vi "Read Analogue.vi"(8 "error in (no error)":errorcluster, 11 "NI Thermo in":refnum<class "NI Thermo.lvclass">) -> (0 "error out":errorcluster, 2 "Waveforms":waveform(dbl)[](array[waveform]), 3 "NI Thermo out":refnum<class "NI Thermo.lvclass">)   [LabVIEW 2025, in "Thermo.lvlib" / "NI Thermo.lvclass"]
uses:
  NI Thermo.lvclass
  NI Thermo.lvclass/NI Thermo.ctl
  Thermo Channel/Thermo Channel.lvclass
  Thermo Channel configuration/Thermo Channel configuration.lvclass
  <vilib>/DAQmx/read.llb/DAQmx Read (Analog 1D DBL NChan 1Samp).vi
  Users/Public/Documents/Sandia National Labs/TSS Plugin/Abstract Engine.lvlibp/Abstract Instrument/Channel.ctl
  Users/Public/Documents/Sandia National Labs/TSS Plugin/Abstract Engine.lvlibp/Abstract Instrument/Abstract Instrument.lvclass
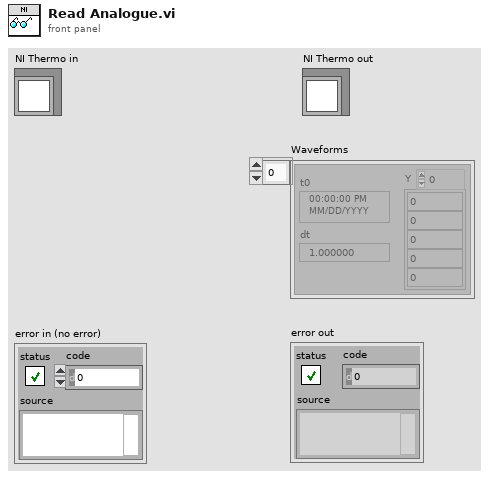
[diagram p1: front panel]
types:
  T1 = typedef "Abstract Engine.lvlibp/Abstract Instrument.lvclass/Channel.ctl" = cluster{"Alias":string, "DataType":enum16{"Anaolg Input", "Waveform"}, "Unit":enum16{"---", "V", "A", "Ohm", "Hz", "uF", "degC", "deg"}, "Upper limit":dbl, "Lower limit":dbl, "Measurement":variant}
  T2 = enum16{"---", "V", "A", "Ohm", "Hz", "uF", "degC", "deg"}
  T3 = typedef "Abstract Engine.lvlibp/Channel configuration.lvclass/Default Channel.ctl" = cluster{"Address":string, "SW Alias":string, "Enabled":bool, "Type":string, "Description":string}
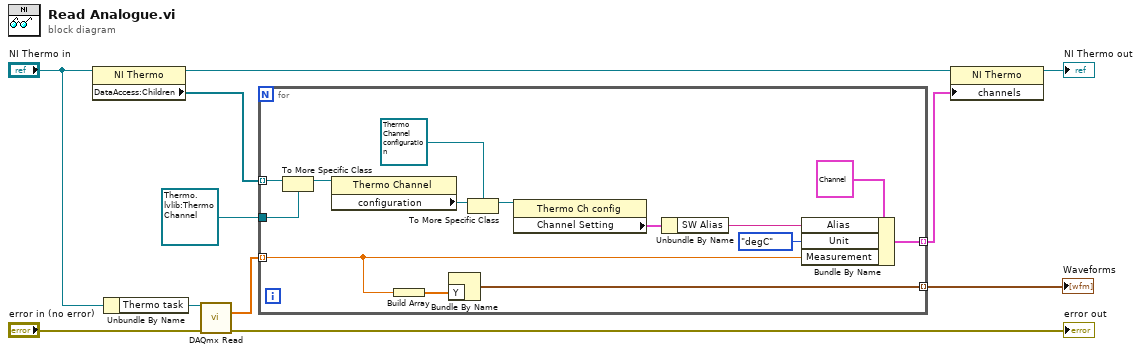
[diagram p0: block diagram]
diagram:
  n1 = property class="NI Thermo"(reference="NI Thermo in") -> (reference out=w7:refnum<class "NI Thermo.lvclass">, "DataAccess:Children"=w6:refnum<data-value>[])  [unwired: 1 in, 1 out]
  n2 = Unbundle By Name("NI Thermo in") -> ("Thermo task"=w8:refnum<k21>)
  n3 = call-poly <vilib>:"DAQmx Read.vi"("task/channels in"=w8, "error in"="error in (no error)") -> ("data"=w4:dbl[], "error out"=→"error out":errorcluster)  [unwired: 11 in, 1 out]
  n4 = for {
    tunnel: w4 -> [w14] mode=indexing
    tunnel: w6 -> [w25] mode=indexing
    tunnel: [w19] -> w2 mode=indexing
    tunnel: refnum<data-value> refnum ("data value reference") -> [w18]
    tunnel: [w12] -> w1 mode=indexing
    n5 = To More Specific Class(target class=w18, reference=w25) -> (specific class reference=w24:refnum<data-value>)  [unwired: 1 in, 1 out]
    n6 = property class="Thermo Channel"(reference=w24) -> ("configuration"=w23:refnum<class "CEF_serializable configuration.lvclass">)  [unwired: 1 in, 2 out]
    n7 = Build Array(w14) -> (w13:dbl[])
    n8 = Bundle By Name("Y"=w13) -> (w12:waveform(dbl))  [unwired: 1 in]
    n9 = To More Specific Class(target class=refnum<class "Thermo Channel configuration.lvclass"> refnum ("Thermo.lvlib:Thermo Ch config"), reference=w23) -> (specific class reference=w22:refnum<class "Thermo Channel configuration.lvclass">)  [unwired: 1 in, 1 out]
    n10 = property class="Thermo Ch config"(reference=w22) -> ("Channel Setting"=w21:T3)  [unwired: 1 in, 2 out]
    n11 = Unbundle By Name(w21) -> ("SW Alias"=w20:string)
    n12 = Bundle By Name(cluster=T1 {"Alias"="ch0", "DataType"=enum."Anaolg Input", "Unit"=enum."V", "Upper limit"=10.0, "Lower limit"=-10.0, "Measurement"=variant} ("Channel"), "Alias"=w20, "Unit"=T2."degC", "Measurement"=w14) -> (w19:T1)
  }
  "Waveforms" <- w1
  n13 = property class="NI Thermo"(reference=w7, "channels"=w2) -> (reference out=→"NI Thermo out":refnum<class "NI Thermo.lvclass">)  [unwired: 1 in, 1 out]
